vi "getModbusConfig.vi"(8 "Error In":errorcluster, 11 "Modbus Config File Path":path) -> (0 "Error Out":errorcluster, 3 "PLC Data":T1={"IP Address"="", "Timeout"=0, "Port [502]"=0, "isSimulation?"=FALSE, "Model Number"=0, "Read Modbus Register"={"Starting Address"=0, "Number of Inputs"=1}, "Individual Address"=[], "Model Changed?"=FALSE, "Models Table"=[], "Status?"=FALSE})   [LabVIEW 2018]
uses:
  controls/modbusData.ctl
  controls/readRegisterModbusCluster.ctl
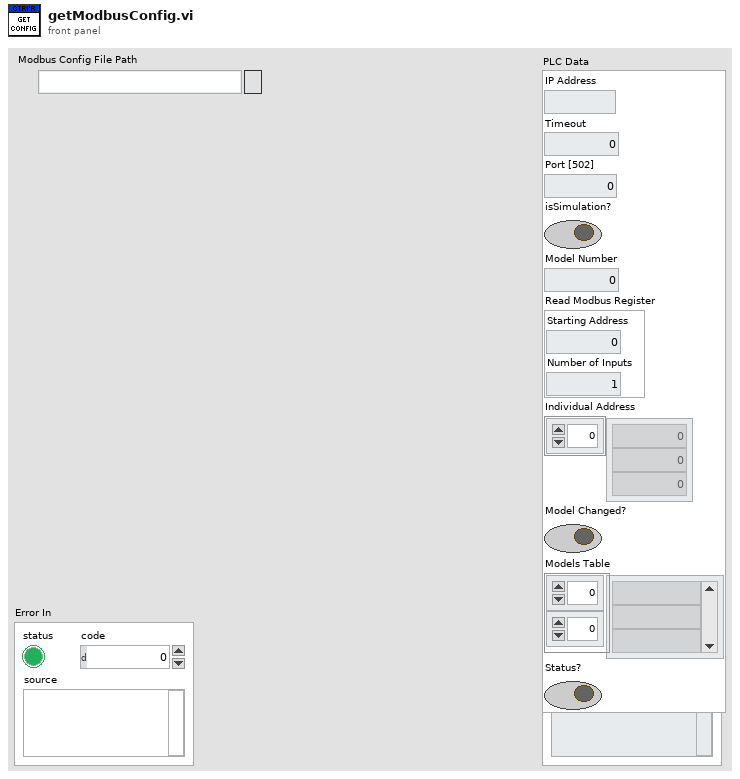
[diagram p1: front panel]
types:
  T1 = typedef "modbusData.ctl" = cluster{"IP Address":string, "Timeout":i32, "Port [502]":u16, "isSimulation?":bool, "Model Number":u16, "Read Modbus Register":T2, "Individual Address":u16[], "Model Changed?":bool, "Models Table":string[][], "Status?":bool}
  T2 = typedef "readRegisterModbusCluster.ctl" = cluster{"Starting Address":u16, "Number of Inputs":u16}
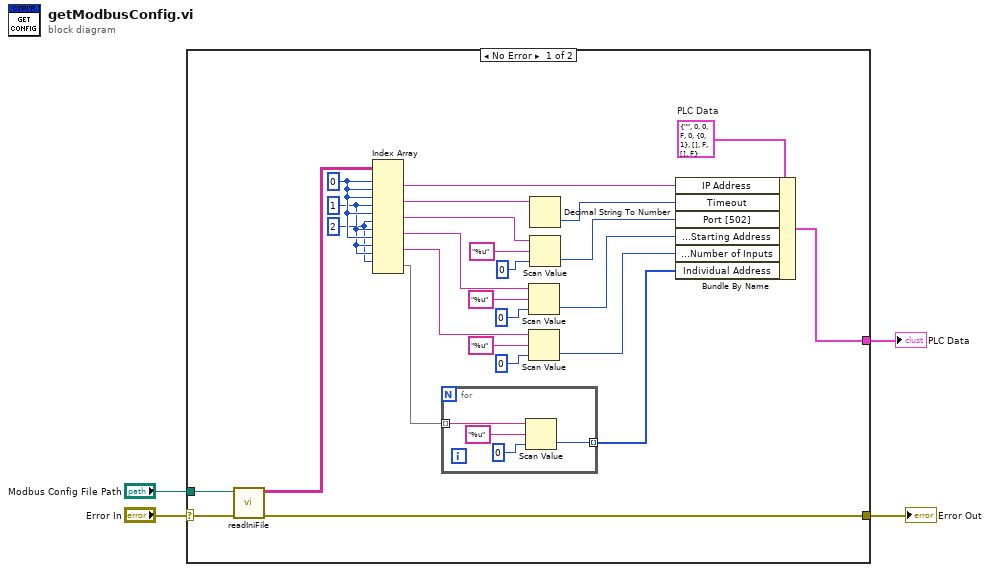
[diagram p0: block diagram]
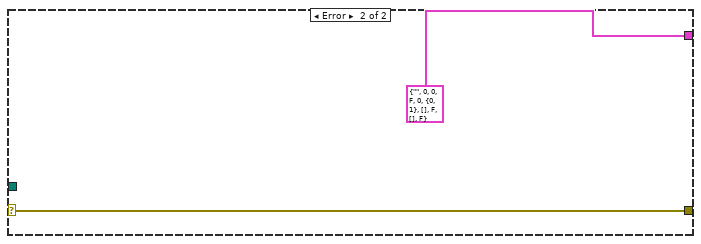
[diagram p2: hidden frame]
diagram:
  n1 = case shown="No Error" "Error In" {
    selector: "Error In" -> [w30 w36]
    tunnel: [w29 w36] -> w3
    tunnel: "Modbus Config File Path" -> [w28 _]
    tunnel: [w20 T1 {"IP Address"="", "Timeout"=0, "Port [502]"=0, "isSimulation?"=FALSE, "Model Number"=0, "Read Modbus Register"={"Starting Address"=0, "Number of Inputs"=1}, "Individual Address"=[], "Model Changed?"=FALSE, "Models Table"=[], "Status?"=FALSE} ("PLC Data")] -> w1
    frame No Error {
      w7 = 2 ("disabled index (col)")
      w8 = 1 ("disabled index (col)")
      w26 = T1 {"IP Address"="", "Timeout"=0, "Port [502]"=0, "isSimulation?"=FALSE, "Model Number"=0, "Read Modbus Register"={"Starting Address"=0, "Number of Inputs"=1}, "Individual Address"=[], "Model Changed?"=FALSE, "Models Table"=[], "Status?"=FALSE}  # PLC Data
      w18 = 0 ("index (row)")
      n2 = call "readIniFile.vi"("Error In"=w30, "File Path Control"=w28) -> ("Error Out"=w29:errorcluster, "Value"=w27:string[][])  [unwired: 8 in]
      n3 = Index Array(array=w27, index (row) #1=w18, index (col) #1=w18, index (row) #2=w18, index (col) #2=w8, index (row) #3=w18, index (col) #3=w7, index (row) #4=w8, index (col) #4=w18, index (row) #5=w8, index (col) #5=w8, index (row) #6=w7) -> (element #1=w25:string, element #2=w24:string, element #3=w22:string, element #4=w14:string, element #5=w10:string, element #6=w6:string[])  [unwired: 1 in]
      n4 = for {
        tunnel: w6 -> [w32] mode=indexing
        tunnel: [w31] -> w5 mode=indexing
        n5 = Scan Value(string=w32, format string="%u", default (0 dbl)=u16 0 ("Port [502]")) -> (value=w31:u16)  [unwired: 1 out]
      }
      n6 = Scan Value(string=w14, format string="%u", default (0 dbl)=u16 0 ("Port [502]")) -> (value=w13:u16)  [unwired: 1 out]
      n7 = Scan Value(string=w10, format string="%u", default (0 dbl)=u16 0 ("Port [502]")) -> (value=w9:u16)  [unwired: 1 out]
      n8 = Decimal String To Number(string=w24) -> (number=w23:i32)  [unwired: 2 in, 1 out]
      n9 = Scan Value(string=w22, format string="%u", default (0 dbl)=u16 0 ("Port [502]")) -> (value=w21:u16)  [unwired: 1 out]
      n10 = Bundle By Name(cluster=w26, "IP Address"=w25, "Timeout"=w23, "Port [502]"=w21, "Read Modbus Register.Starting Address"=w13, "Read Modbus Register.Number of Inputs"=w9, "Individual Address"=w5) -> (w20:T1)
    }
    frame Error {
    }
  }
  "Error Out" <- w3
  "PLC Data" <- w1
